vi "ResizeCore_ARGB.vi"(7 "OpenCV Interpolation Flag":T1, 8 "error in (no error)":errorcluster, 9 "Retain Data?":bool, 10 "ImageSize":T2, 11 "ARGB Image":refnum<data-value>) -> (0 "error out":errorcluster)   [LabVIEW 2020, in "g_ar_toolkit.lvlib"]
uses:
  g_ar_toolkit.lvlib
  Image Size Cluster.ctl
  OpenCV Interpolation Enum.ctl
  g_ar_toolkit.32.dll
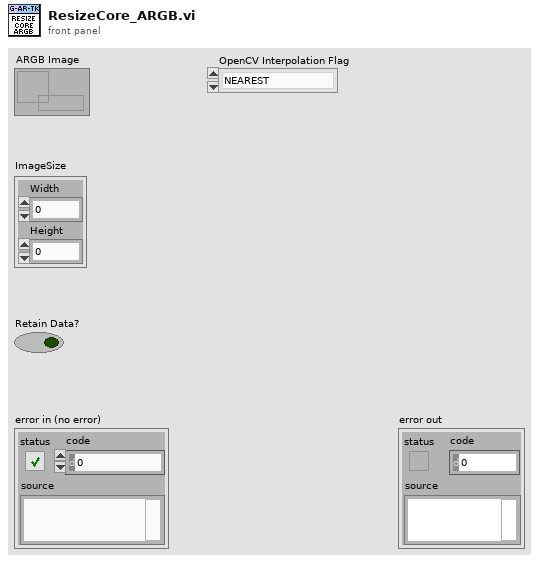
[diagram p1: front panel]
types:
  T1 = typedef "g_ar_toolkit.lvlib/OpenCV Interpolation Enum.ctl" = enum16{"NEAREST", "LINEAR", "CUBIC", "AREA", "LANCZOS", "LINEAR_EXACT", "NEAREST_EXACT", "MAX"}
  T2 = typedef "g_ar_toolkit.lvlib/Image Size Cluster.ctl" = cluster{"Width":u16, "Height":u16}
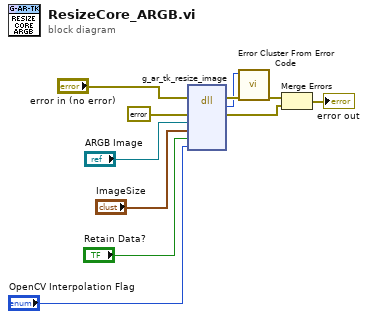
[diagram p0: block diagram]
diagram:
  n1 = dll-call lib="C:/serenial/libraries/g-augmented-reality-toolkit/LabVIEW/g_ar_toolkit/g_ar_toolkit.*.*" fn="g_ar_tk_resize_image"(error in="error in (no error)", "error_cluster"=errorcluster {"status"=FALSE, "code"=0, "source"=""} ("error constant"), "EDVR"="ARGB Image", "ImageSize"="ImageSize", "retain_data"="Retain Data?", "interpolation_mode"="OpenCV Interpolation Flag") -> (error out=w8:errorcluster, "MgErr"=w7:i32, "error_cluster"=w1:errorcluster)  [unwired: 6 in, 1 out]
  n2 = call <vilib>:"Error Cluster From Error Code.vi"("error in (no error)"=w8, "error code (0)"=w7) -> ("error out"=w5:errorcluster)  [unwired: 7 in]
  n3 = Merge Errors(w5, w1) -> (→"error out":errorcluster)
